vi "TakeVData_CO.vi"(0 "Sensor":u16(ring)=1 items=["No1"=1, "No 2"=2, "No 3"=3, "No 4"=4], 2 "Measurement wait time (ms)":dbl=300.0, 3 "Setpoint temperature (K)":dbl=50.0 format="%.3f", 4 "Allowable deviation (K)":dbl=0.005 format="%.4f", 5 "Number of voltage measurements\nbetween temperature check":dbl=10.0, 6 "Temperature Controller GPIB address":string="15", 8 "DMM (to sample) GPIB address":string="11", 10 "DMM2 GPIB address":string="22", 15 "Cutoff (mV)":dbl=1.0 format="%.2f") -> (7 "Mean Temp (C)":dbl=50.00011818181817 format="%.6f", 9 "Temp error (C)":dbl=9.107990624382646e-05 format="%.6f", 11 "Voltage error 2 (V)":dbl=0.00181175202707556 format="%.6f", 13 "Mean Voltage 2 (V)":dbl=5.678862454545454 format="%.6f", 16 "Temperature stable?":bool=TRUE, 17 "Mean Voltage 1 (V)":dbl=4.278487636363637 format="%_4e", 18 "Voltage error 1 (V)":dbl=0.004019221765689146 format="%.6f", 19 "Number of measurements":dbl=110.0)   [LabVIEW 2014]
uses:
  <vilib>/Analysis/NI_AALBase.lvlib
panel:
  out "Current mean":dbl=4.278487636363637 format="%_4e"
  out "XY Graph":T1(graph)={"X Values"=[4.1453515, 4.1701545, 4.1949575, 4.2197605000000005, 4.2445635, 4.2693665, 4.2941695, 4.3189725, 4.3437755000000005, 4.3685785], "Histogram: h(x)"=[1, 1, 3, 9, 16, 29, 24, 17, 6, 4]}
  out "Waveform Graph":dbl[](graph)=[4.27891, 4.28936, 4.28463, 4.29806, 4.22459, 4.25078, 4.21523, 4.2593, 4.26288, 4.29395, 4.36497, 4.27288, 4.24771, 4.33354, 4.23355, 4.25705, 4.21775, 4.30322, 4.27666, 4.25329, 4.24555, 4.19811, 4.26127, 4.30122, 4.29745, 4.31371, 4.32614, 4.31055, 4.26262, 4.30773, 4.27151, 4.21924, 4.28738, 4.28483, 4.3166, 4.25723, 4.21226, 4.34617, 4.20113, 4.23813, 4.24504, 4.29924, 4.27879, 4.28236, 4.23821, 4.36495, 4.28611, 4.32455, 4.27014, 4.17858, 4.33211, 4.25687, 4.33623, 4.25839, 4.32694, 4.36634, 4.29566, 4.13295, 4.35364, 4.32, 4.26607, 4.26596, 4.27724, 4.33095, 4.2826, 4.1969, 4.27606, 4.28026, 4.31659, 4.32486, 4.34038, 4.22827, 4.28215, 4.27773, 4.32973, 4.27652, 4.27319, 4.24642, 4.25515, 4.28267, 4.31099, 4.25545, 4.29572, 4.25074, 4.29203, 4.26923, 4.30546, 4.27706, 4.32856, 4.20922, 4.30972, 4.25705, 4.27274, 4.30608, 4.2778, 4.29801, 4.38098, 4.26683, 4.23028, 4.28822, 4.21281, 4.25234, 4.29412, 4.2609, 4.25508, 4.27464, 4.24901, 4.31814, 4.31046, 4.29003]
  out "Loop No.":dbl=10.0 format="%#_4f"
  out "Current precision":dbl=1064.5064855310457 format="%_6f"
  out "Current error (mV)":dbl=0.004019221765689146 format="%_4e"
  in  "Precision":dbl=1000.0 format="%.2f"
  # "For high precision,\n0.15 works well."
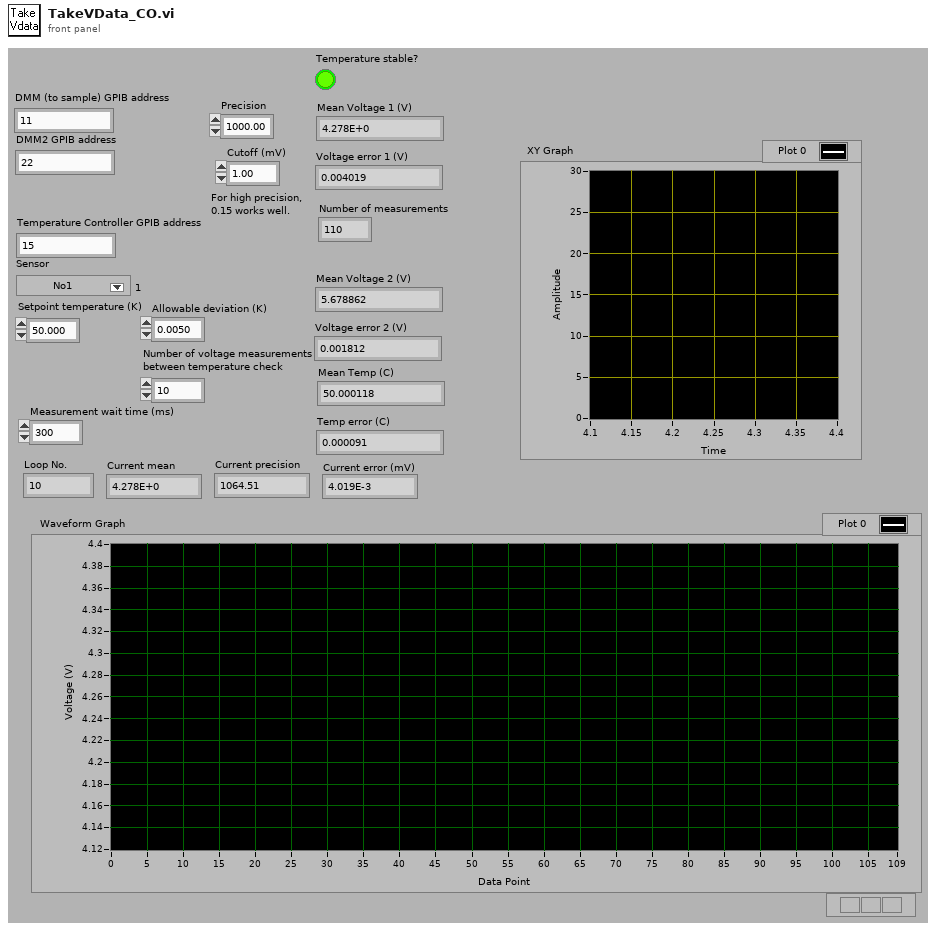
[diagram p1: front panel]
types:
  T1 = cluster{"X Values":dbl[], "Histogram: h(x)":i32[]}
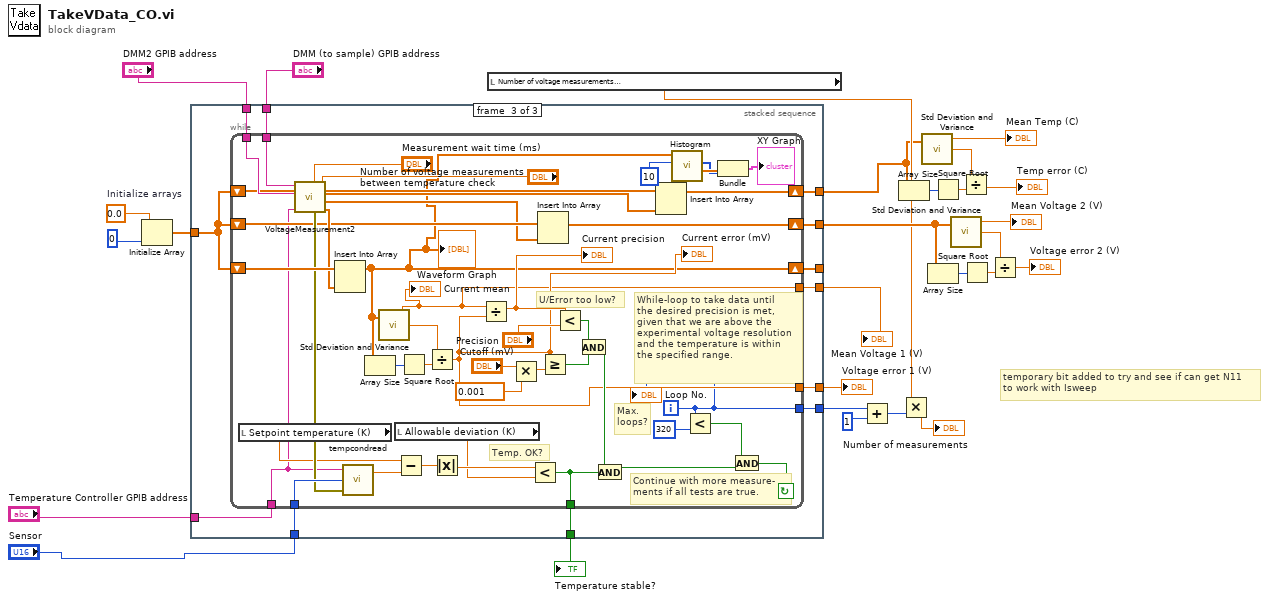
[diagram p0: block diagram]
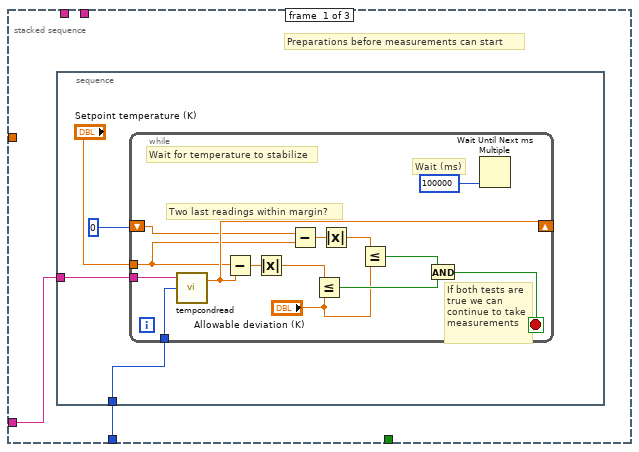
[diagram p2: hidden frame]
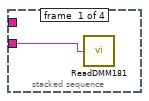
[diagram p4: hidden frame]
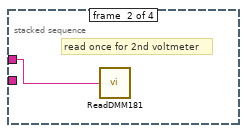
[diagram p5: hidden frame]
diagram:
  w25 = 0.0  # Initialize arrays
  # "temporary bit added to try and see if can get N11\nto work with Isweep"
  n1 = Initialize Array(w25, 0) -> (w24:dbl[])
  n2 = stacked-sequence {
    tunnel: "DMM (to sample) GPIB address" -> [_ w49 w63]
    tunnel: w24 -> [_ _ w53]
    tunnel: "Sensor" -> [w28 _ w62]
    tunnel: "Temperature Controller GPIB address" -> [w29 _ w61]
    tunnel: [_ _ w60] -> w22
    tunnel: [_ _ w59] -> _
    tunnel: [_ _ w58] -> w20
    tunnel: [_ _ w57] -> w17
    tunnel: [_ _ w56] -> w8
    tunnel: "DMM2 GPIB address" -> [_ w48 w55]
    tunnel: [_ _ w54] -> w12
    tunnel: [_ _ w52] -> w2
    frame #0 {
      # "Preparations before measurements can start"
      n3 = stacked-sequence {
        tunnel: w29 -> [w33]
        tunnel: w28 -> [w32]
        frame #0 {
          n4 = while {
            shift-left: 0 -> [w35]
            shift-right: [w37] -> _
            tunnel: w32 -> [w41]
            tunnel: w33 -> [w45]
            tunnel: "Setpoint temperature (K)" -> [w36]
            stop <- w43 stop-if-true
            # "If both tests are\ntrue we can\ncontinue to take\nmeasurements"
            # "Two last readings within margin?"
            # "Wait for temperature to stabilize"
            # "Wait (ms)"
            n5 = call "tempcondread.vi"("Ring"=w41, "GPIB Address"=w45) -> ("Temperature"=w37:dbl)  [unwired: 1 in, 1 out]
            n6 = Subtract(x=w36, y=w37) -> (x-y=w46:dbl)
            n7 = Absolute Value(x=w46) -> (abs(x)=w42:dbl)
            n8 = Subtract(x=w35, y=w36) -> (x-y=w40:dbl)
            n9 = Less Or Equal?(x=w42, y="Allowable deviation (K)") -> (x <= y?=w44:bool)
            n10 = Absolute Value(x=w40) -> (abs(x)=w39:dbl)
            n11 = Less Or Equal?(x=w39, y="Allowable deviation (K)") -> (x <= y?=w38:bool)
            n12 = And(x=w38, y=w44) -> (x .and. y?=w43:bool)
            n13 = Wait Until Next ms Multiple(millisecond multiple=100000) -> ()  [unwired: 1 out]
          }
        }
      }
    }
    frame #1 {
      n14 = stacked-sequence {
        tunnel: w49 -> [w50 _ _ _]
        tunnel: w48 -> [_ w51 _ _]
        frame #0 {
          n15 = call "ReadDMM181.vi"("DMM GPIB Address"=w50) -> ()  [unwired: 1 out]
        }
        frame #1 {
          # "read once for 2nd voltmeter"
          n16 = call "ReadDMM181.vi"("DMM GPIB Address"=w51) -> ()  [unwired: 1 out]
        }
        frame #2 {
          # "read once for 3rd voltmeter"
        }
        frame #3 {
        }
      }
    }
    frame #2 {
      n17 = while {
        shift-left: w53 -> [w79]
        shift-right: [w78] -> w52
        shift-left: w53 -> [w86]
        shift-right: [w87] -> w54
        tunnel: w55 -> [w90]
        tunnel: [w65] -> w56
        tunnel: [w72] -> w57
        tunnel: [w71] -> w58
        tunnel: [w103] -> w60
        tunnel: w61 -> [w64]
        tunnel: w62 -> [w105]
        shift-left: w53 -> [w102]
        shift-right: [w70] -> w59
        tunnel: w63 -> [w89]
        i -> [w71]
        stop <- w97 continue-if-true
        # "U/Error too low?"
        # "Max.\nloops?"
        # "Continue with more measure-\nments if all tests are true."
        # "While-loop to take data until\nthe desired precision is met,\ngiven that we are above the\nexperimental voltage resolution\nand the temperature is within\nthe specified range."
        # "Temp. OK?"
        n18 = local read "Setpoint temperature (K)"() -> (w83:dbl)
        n19 = call "VoltageMeasurement2.vi"("Number of measurements"="Number of voltage measurements\nbetween temperature check", "Measurement wait time (ms)"="Measurement wait time (ms)", "Temp Controller address"=w64, "DMM2 GPIB address"=w90, "DMM GPIB address"=w89) -> ("Voltage 1 (V)"=w88:dbl[], "Voltage 2 (V)"=w85:dbl[], "Temperature (C)"=w77:dbl[], "error out"=w101:errorcluster)  [unwired: 3 in]
        n20 = Insert Into Array(array=w102, new element=w88) -> (w70:dbl[])  [unwired: 1 in]
        "Waveform Graph" <- w70
        n21 = call "tempcondread.vi"("error in"=w101, "Ring"=w105, "GPIB Address"=w64) -> ("Temperature"=w106:dbl)  [unwired: 1 out]
        n22 = Array Size(array=w70) -> (size(s)=w93:i32)
        n23 = call <vilib>:"Std Deviation and Variance.vi"("X"=w70) -> ("mean"=w65:dbl, "standard deviation"=w92:dbl)  [unwired: 1 in, 1 out]
        "Current mean" <- w65
        n24 = local read "Allowable deviation (K)"() -> (w81:dbl)
        n25 = Subtract(x=w83, y=w106) -> (x-y=w107:dbl)
        n26 = Square Root(x=w93) -> (sqrt(x)=w91:dbl)
        n27 = Divide(x=w92, y=w91) -> (x/y=w72:dbl)
        "Current error (mV)" <- w72
        n28 = Absolute Value(x=w107) -> (abs(x)=w104:dbl)
        n29 = Divide(x=w65, y=w72) -> (x/y=w73:dbl)
        "Current precision" <- w73
        n30 = Multiply(x="Cutoff (mV)", y=0.001) -> (x*y=w74:dbl)
        n31 = Less?(x=w104, y=w81) -> (x < y?=w103:bool)
        n32 = Insert Into Array(array=w86, new element=w85) -> (w87:dbl[])  [unwired: 1 in]
        n33 = Greater Or Equal?(x=w72, y=w74) -> (x >= y?=w96:bool)
        n34 = Less?(x=w73, y="Precision") -> (x < y?=w95:bool)
        n35 = And(x=w95, y=w96) -> (x .and. y?=w94:bool)
        n36 = And(x=w94, y=w103) -> (x .and. y?=w99:bool)
        n37 = Insert Into Array(array=w79, new element=w77) -> (w78:dbl[])  [unwired: 1 in]
        n38 = call <vilib>:"Histogram.vi"("intervals"=10, "X"=w70) -> ("X Values"=w67:dbl[], "Histogram: h(x)"=w66:i32[])  [unwired: 6 in, 2 out]
        n39 = Less?(x=w71, y=320) -> (x < y?=w98:bool)
        n40 = Bundle("X Values"=w67, "Histogram: h(x)"=w66) -> (→"XY Graph":T1)  [unwired: 1 in]
        n41 = And(x=w98, y=w99) -> (x .and. y?=w97:bool)
        "Loop No." <- w71
      }
    }
  }
  "Temperature stable?" <- w22
  "Voltage error 1 (V)" <- w17
  "Mean Voltage 1 (V)" <- w8
  n42 = local read "Number of voltage measurements\nbetween temperature check"() -> (w9:dbl)
  n43 = Add(x=w20, y=1) -> (x+y=w18:i32)
  n44 = Array Size(array=w2) -> (size(s)=w5:i32)
  n45 = Multiply(x=w9, y=w18) -> (x*y=→"Number of measurements":dbl)
  n46 = call <vilib>:"Std Deviation and Variance.vi"("X"=w2) -> ("mean"=→"Mean Temp (C)":dbl, "standard deviation"=w6:dbl)  [unwired: 1 in, 1 out]
  n47 = Array Size(array=w12) -> (size(s)=w13:i32)
  n48 = Square Root(x=w5) -> (sqrt(x)=w7:dbl)
  n49 = call <vilib>:"Std Deviation and Variance.vi"("X"=w12) -> ("mean"=→"Mean Voltage 2 (V)":dbl, "standard deviation"=w14:dbl)  [unwired: 1 in, 1 out]
  n50 = Divide(x=w6, y=w7) -> (x/y=→"Temp error (C)":dbl)
  n51 = Square Root(x=w13) -> (sqrt(x)=w15:dbl)
  n52 = Divide(x=w14, y=w15) -> (x/y=→"Voltage error 2 (V)":dbl)
